vi "cdex_Pitch PID.vi"(9 "pitch speed":dbl, 11 "pitch set point":dbl) -> (2 "Output (u)":dbl)   [LabVIEW 2015]
uses:
  <vilib>/Simulation/Implementation/Shared/SIMSCR Execution Mode.ctl
  <vilib>/Simulation/Scripting/Companion Diagram/SimConfigNode/SimParams.ctl
  <vilib>/Simulation/Scripting/Companion Diagram/SimConfigNode/_simSolvers.ctl
  <vilib>/Simulation/Param Hierarchy/Typedefs/SIMPH Param Control Actions.ctl
  <vilib>/Simulation/Implementation/Shared/SIM limit type.ctl
  <vilib>/Simulation/Implementation/Shared/NILVSim_ParamChanged.vi
  <vilib>/Simulation/Implementation/Shared/NILVSIM_BeginStep.vi
  <vilib>/Simulation/SignalArithmetic/Implementation/NILVSim Gain.llb/SIM Gain (scalar).vi
  <vilib>/Simulation/ContinuousLinear/Implementation/NILVSim Integrator new.llb/SIM Integrator distributor (scalar).vi
  <vilib>/Simulation/ContinuousLinear/Implementation/NILVSim Integrator new.llb/SIM Integrator collector (scalar).vi
  <vilib>/Simulation/Nonlinear/Implementation/NILVSim Saturation.llb/SIM Saturation (scalar).vi
  <vilib>/Simulation/Implementation/Shared/NILVSim_Manager.vi
  <vilib>/Utility/error.llb/Clear Errors.vi
  <vilib>/Simulation/Implementation/Shared/NILVSim_FinalizeModel.vi
  <vilib>/Simulation/Implementation/Shared/SIM Unbundle Sim Info.vi
  <vilib>/Simulation/Implementation/Shared/SIMSH Read Queue.vi
  3DHe_Global.vi
  <vilib>/Simulation/Implementation/Shared/NILVSim_Initialize.vi
  <vilib>/Simulation/Utility/Implementation/NILVSim Get Time and IsAcceptedStep.vi
  <vilib>/Simulation/Implementation/Shared/NILVSim_GetModelError.vi
  <vilib>/Simulation/Implementation/Shared/SIM SimErrorHandler.vi
  <vilib>/Simulation/Implementation/Shared/SIM Bundle Sim Info.vi
  <vilib>/Simulation/Scripting/Companion Diagram/SimConfigNode/SimDog.xnode
  <vilib>/Simulation/Implementation/XNodeFramework/SimXNode/SimX.xnode
  <vilib>/Simulation/ContinuousLinear/Implementation/NILVSim Integrator new.llb/SIM Integrator (scalar).vi
  <vilib>/Simulation/Implementation/Shared/NI_SIM_Implementation.lvlib
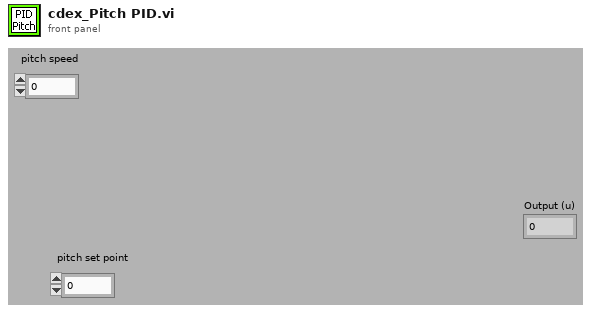
[diagram p1: front panel]
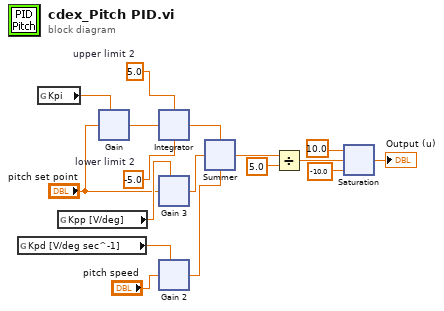
[diagram p0: block diagram]
diagram:
  w12 = -5.0  # lower limit 2
  w13 = 5.0  # upper limit 2
  n1 = global read "3DHe_Global.vi" "Kpd [V/deg sec^-1]"() -> (w3:dbl)
  n2 = global read "3DHe_Global.vi 2" "Kpi"() -> (w4:dbl)
  n3 = global read "3DHe_Global.vi 3" "Kpp [V/deg]"() -> (w5:dbl)
  n4 = xnode ("Gain")("gain"=w4, "input"="pitch set point") -> ("output"=w16:dbl)  [unwired: 2 in]
  n5 = xnode ("Integrator")("upper limit"=w13, "input"=w16, "lower limit"=w12) -> ("output"=w15:dbl)  [unwired: 7 in, 2 out]
  n6 = xnode ("Gain 3")("gain"=w5, "input"="pitch set point") -> ("output"=w17:dbl)  [unwired: 2 in]
  n7 = xnode ("Gain 2")("gain"=w3, "input"="pitch speed") -> ("output"=w14:dbl)  [unwired: 2 in]
  n8 = xnode ("Summer")("Operand1"=w15, "Operand2"=w17, "Operand3"=w14) -> ("Result"=w10:dbl)
  n9 = Divide(x=w10, y=5.0 ("Constant")) -> (x/y=w9:dbl)
  n10 = xnode ("Saturation")("upper limit"=10.0, "input"=w9, "lower limit"=-10.0) -> ("output"=→"Output (u)":dbl)  [unwired: 2 in]
